vi "StopForLog.vi"() -> ()   [LabVIEW 2014]
panel:
  in  "StopForLog":bool
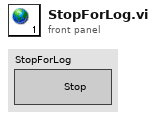
[diagram p1: front panel]
diagram:
